vi "Configure Pulse.vi"(0 "VISA resource name":refnum<visa-resource-name>, 1 "Pulse Count (1)":dbl=1.0, 5 "Pulse Duty Cycle (50%)":i32=50, 7 "Pulse Hold Type (0:Width)":u32(ring) items=["Width", "Duty Cycle"], 9 "Pulse Period (0.03333 Sec)":dbl=0.03333, 11 "error in (no error)":errorcluster, 12 "Pulse Width (0.01667 Sec)":dbl=0.01667 format="%#_8g", 13 "Enable/Disable Control":T1={"Enable Duty Cycle (T: Enable)"=TRUE, "Enable Period (T: Enable)"=TRUE, "Enable Width (T: Enable)"=TRUE}) -> (4 "VISA resource name out":refnum<visa-resource-name>, 15 "error out":errorcluster)   [LabVIEW 2010, in "California Instruments iX Series.lvlib"]
doc: "Configures the generation of output pulses. The duty cycle, hold type, period and width controls are coupled, which means that the values set by any one of these commands can affect the settings of the other."
uses:
  <instrlib>/California Instruments iX Series/California Instruments iX Series.lvlib
panel:
  # "Refer to Block Diagram for description on how duty cycle, period and width are affected when one, two or all three parameters are set."
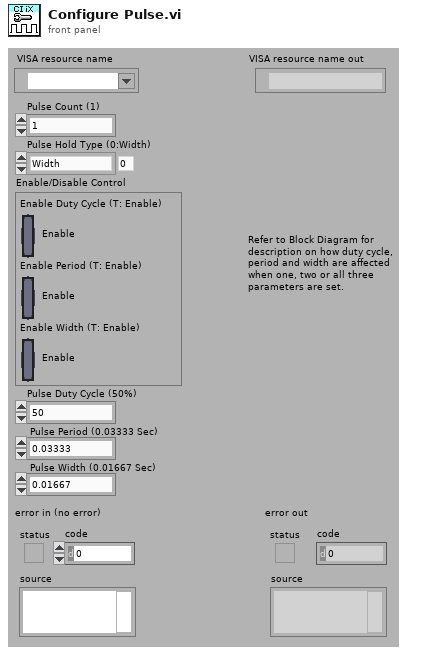
[diagram p1: front panel]
types:
  T1 = cluster{"Enable Duty Cycle (T: Enable)":bool, "Enable Period (T: Enable)":bool, "Enable Width (T: Enable)":bool}
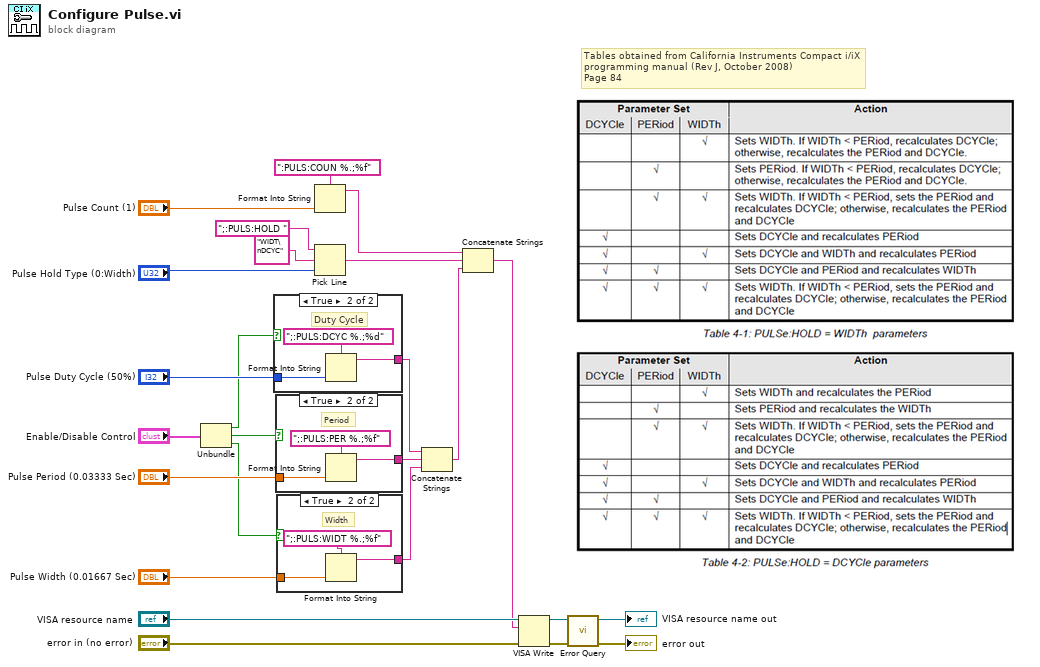
[diagram p0: block diagram]
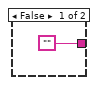
[diagram p2: hidden frame]
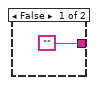
[diagram p3: hidden frame]
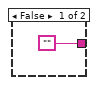
[diagram p4: hidden frame]
diagram:
  # "Tables obtained from California Instruments Compact i/iX programming manual (Rev J, October 2008)\nPage 84"
  n1 = Unbundle("Enable/Disable Control") -> ("Enable Duty Cycle (T: Enable)"=w4:bool, "Enable Period (T: Enable)"=w3:bool, "Enable Width (T: Enable)"=w2:bool)
  n2 = case shown="True" w4 {
    tunnel: "Pulse Duty Cycle (50%)" -> [_ w29]
    tunnel: ["" w27] -> w9
    frame False {
    }
    frame True {
      # "Duty Cycle"
      n3 = Format Into String(format string=";:PULS:DCYC %.;%d", w29) -> (resulting string=w27:string)  [unwired: 2 in, 1 out]
    }
  }
  n4 = case shown="True" w3 {
    tunnel: "Pulse Period (0.03333 Sec)" -> [_ w33]
    tunnel: ["" w31] -> w8
    frame False {
    }
    frame True {
      # "Period"
      n5 = Format Into String(format string=";:PULS:PER %.;%f", w33) -> (resulting string=w31:string)  [unwired: 2 in, 1 out]
    }
  }
  n6 = case shown="True" w2 {
    tunnel: "Pulse Width (0.01667 Sec)" -> [_ w37]
    tunnel: ["" w35] -> w7
    frame False {
    }
    frame True {
      # "Width"
      n7 = Format Into String(format string=";:PULS:WIDT %.;%f", w37) -> (resulting string=w35:string)  [unwired: 2 in, 1 out]
    }
  }
  n8 = Format Into String(format string=":PULS:COUN %.;%f", "Pulse Count (1)") -> (resulting string=w14:string)  [unwired: 2 in, 1 out]
  n9 = Pick Line(string ("")=";:PULS:HOLD ", multi-line string="WIDT\nDCYC", line index="Pulse Hold Type (0:Width)") -> (output string=w13:string)
  n10 = Concatenate Strings(w9, w8, w7) -> (w6:string)
  n11 = Concatenate Strings(w14, w13, w6) -> (w1:string)
  n12 = VISA Write(VISA resource name="VISA resource name", write buffer=w1, error in (no error)="error in (no error)") -> (VISA resource name out=w23:refnum<visa-resource-name>, error out=w22:errorcluster)  [unwired: 1 out]
  n13 = call <instrlib>:"Error Query.vi"("error in (no error)"=w22, "VISA resource name"=w23) -> ("error out"=→"error out":errorcluster, "VISA resource name out"=→"VISA resource name out":refnum<visa-resource-name>)  [unwired: 6 in, 2 out]
